vi "Initialize.vi"(0 "VISA resource name":refnum<visa-resource-name>, 1 "Error Queue Option":enum16{"Clear Error Queue", "Error Query"}(ring), 5 "RS-232 Settings":T1={"Read Term Char"=enum."CR", "Baud Rate"=enum."19200", "Flow Control\n(XON / XOFF)"=enum."Off"}, 7 "Instrument Type":T2=enum."KE6221", 11 "error in (no error)":errorcluster, 12 "ID Query? (T)":bool=TRUE, 13 "Reset? (T)":bool=TRUE) -> (4 "VISA resource name out":refnum<visa-resource-name>, 15 "error out":errorcluster)   [LabVIEW 2016, in "Keithley 622x.lvlib"]
doc: "Establishes communication with the instrument and optionally performs an instrument identification query and/or an instrument reset. Therefore, call this VI before calling other instrument driver VIs for this instrument. Generally, you need to call the Initialize VI only once at the beginning of an application."
uses:
  Keithley 622x.lvlib
  Utility/Typedefs/KE622x -- Instrument Type.ctl
  Utility/Typedefs/KE622x -- Serial Port Settings.ctl
panel:
  # "(c) 2010 Keithley Instruments.  ALL RIGHTS RESERVED."
  # "Serial settings must match those on the physical instrument.  Hardware flow control is not supported, but software flow control is (XON/XOFF)."
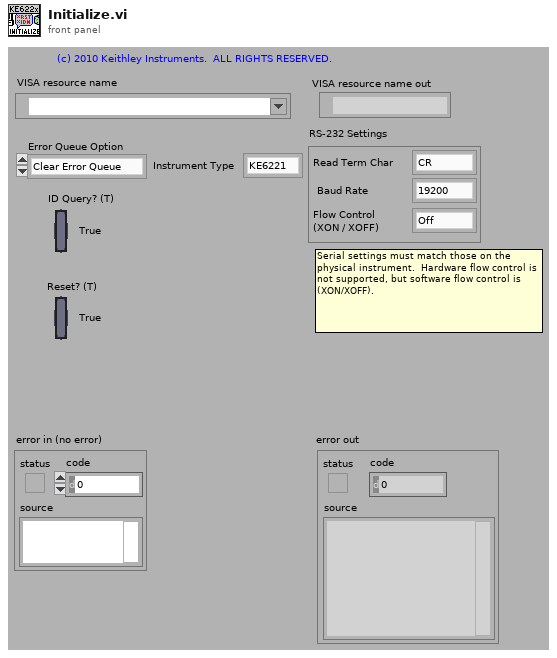
[diagram p1: front panel]
types:
  T1 = typedef "Keithley 622x.lvlib/KE622x -- Serial Port Settings.ctl" = cluster{"Read Term Char":enum16{"CR", "LF", "CR + LF", "LF + CR"}, "Baud Rate":enum16{"300", "600", "1200", "2400", "4800", "9600", "19200", "38400", "57600", "115200"}, "Flow Control\n(XON / XOFF)":enum16{"Off", "On"}}
  T2 = typedef "Keithley 622x.lvlib/KE622x -- Instrument Type.ctl" = enum16{"KE6220", "KE6221"}
  T3 = enum16{"300", "600", "1200", "2400", "4800", "9600", "19200", "38400", "57600", "115200"}
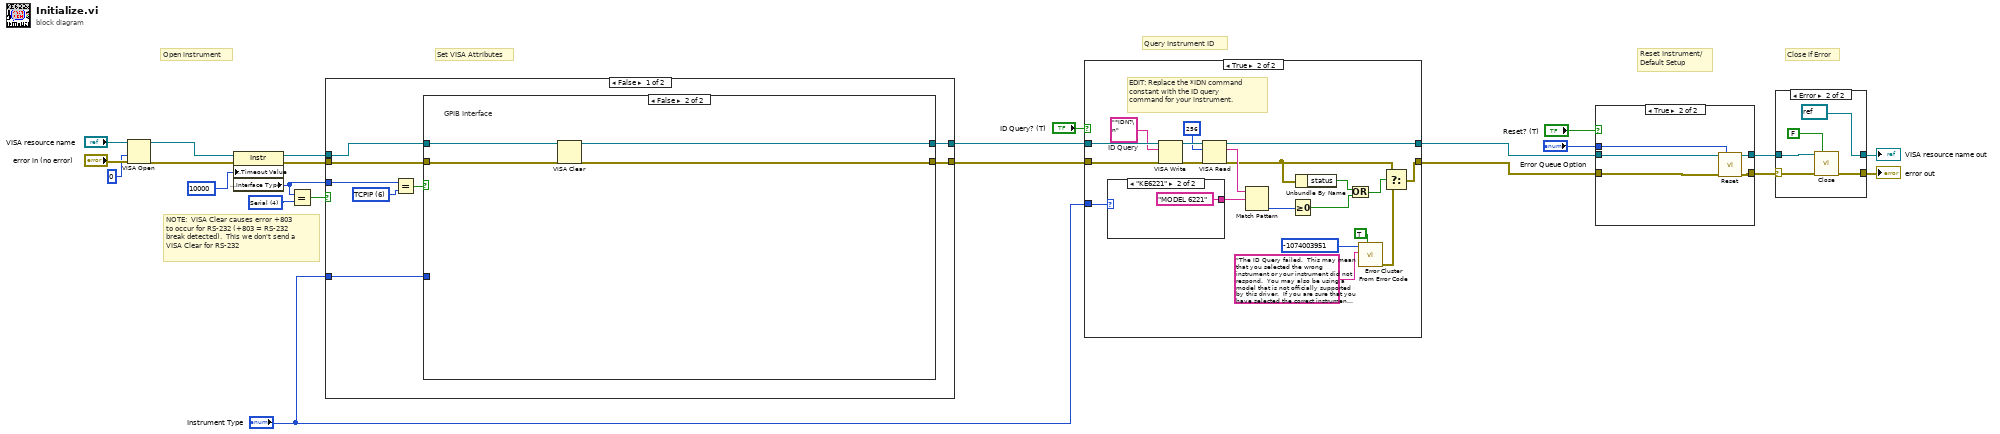
[diagram p0: block diagram]
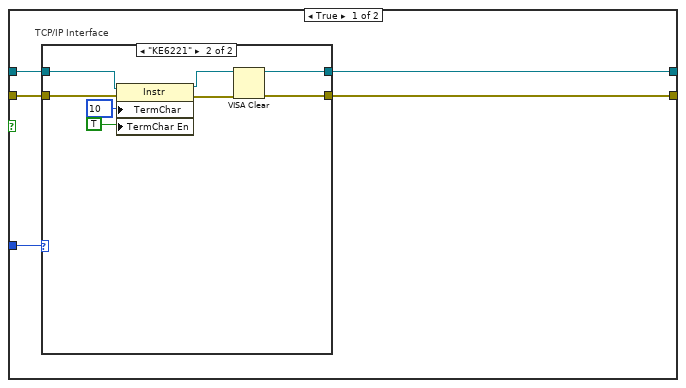
[diagram p2: hidden frame]
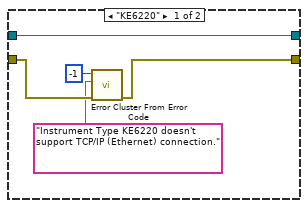
[diagram p3: hidden frame]
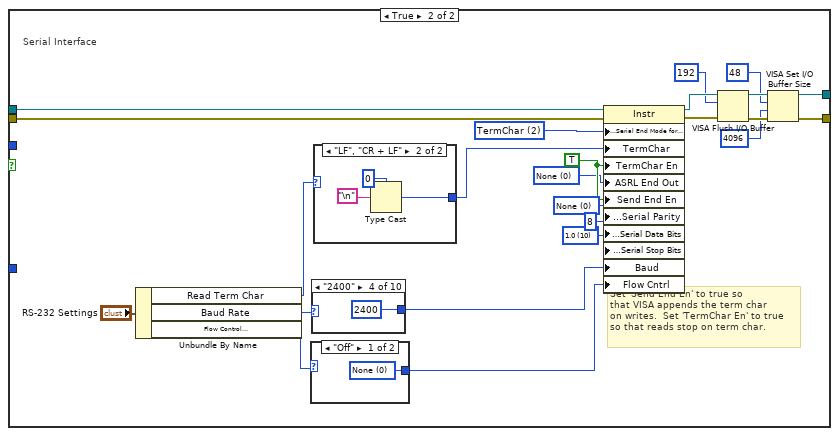
[diagram p4: hidden frame]
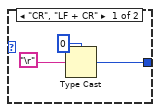
[diagram p5: hidden frame]
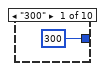
[diagram p6: hidden frame]
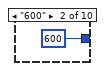
[diagram p7: hidden frame]
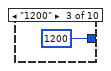
[diagram p8: hidden frame]
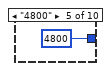
[diagram p9: hidden frame]
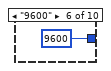
[diagram p10: hidden frame]
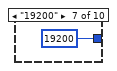
[diagram p11: hidden frame]
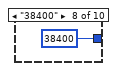
[diagram p12: hidden frame]
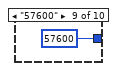
[diagram p13: hidden frame]
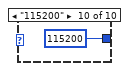
[diagram p14: hidden frame]
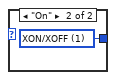
[diagram p15: hidden frame]
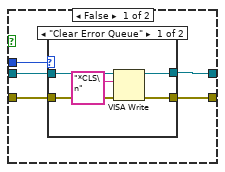
[diagram p17: hidden frame]
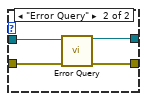
[diagram p18: hidden frame]
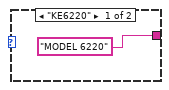
[diagram p20: hidden frame]
diagram:
  w11 = u16 4 items=["GPIB"=1, "VXI"=2, "GPIB-VXI"=3, "Serial"=4, "PXI"=5, "TCPIP"=6, "USB"=7] ("Interface Information:Interface Type")
  # "NOTE:  VISA Clear causes error +803\nto occur for RS-232 (+803 = RS-232\nbreak detected).  This we don't send a\nVISA Clear for RS-232"
  # "Set VISA Attributes"
  # "Close if Error"
  # "Query Instrument ID"
  # "Reset Instrument/\nDefault Setup"
  # "Open instrument"
  n1 = VISA Open(access mode=u32 0, error in (no error)="error in (no error)", VISA resource name="VISA resource name") -> (VISA resource name=w5:refnum<visa-resource-name>, error out=w4:errorcluster)  [unwired: 2 in]
  n2 = property class="Instr"(reference=w5, error in=w4, "General Settings:Timeout Value"=u32 10000) -> (reference out=w14:refnum<visa-resource-name>, error out=w13:errorcluster, "Interface Information:Interface Type"=w2:u16)
  n3 = Equal?(x=w2, y=w11) -> (x = y?=w12:bool)
  n4 = case shown="False" w12 {
    tunnel: [w28 w74] -> w16
    tunnel: [w29 w71] -> w15
    tunnel: w14 -> [w30 w76]
    tunnel: w13 -> [w31 w77]
    tunnel: w2 -> [w27 _]
    tunnel: "Instrument Type" -> [w24 _]
    frame False {
      w26 = u16 6 items=["GPIB"=1, "VXI"=2, "GPIB-VXI"=3, "Serial"=4, "PXI"=5, "TCPIP"=6, "USB"=7] ("Interface Information:Interface Type")
      n5 = Equal?(x=w27, y=w26) -> (x = y?=w25:bool)
      n6 = case shown="False" w25 {
        tunnel: w31 -> [w33 w50]
        tunnel: w30 -> [w34 w51]
        tunnel: [w36 w53] -> w29
        tunnel: [w35 w52] -> w28
        tunnel: w24 -> [w32 _]
        frame True {
          # "TCP/IP Interface"
          n7 = case shown="\"KE6221\"" w32 {
            tunnel: [w37 w49] -> w36
            tunnel: [w41 w48] -> w35
            tunnel: w34 -> [w41 w47]
            tunnel: w33 -> [w40 w44]
            frame "KE6220" {
              n8 = call <vilib>:"Error Cluster From Error Code.vi"("error in (no error)"=w40, "error message (\"\")"="Instrument Type KE6220 doesn't support TCP/IP (Ethernet) connection." ("error message (\"\")"), "error code (0)"=-1) -> ("error out"=w37:errorcluster)  [unwired: 6 in]
            }
            frame "KE6221" {
              n9 = property class="Instr"(reference=w47, error in=w44, "TermChar"=u8 10 ("Message Based Settings:Termination Character"), "TermChar En"=TRUE ("Message Based Settings:Termination Character Enable")) -> (reference out=w42:refnum<visa-resource-name>, error out=w43:errorcluster)
              n10 = VISA Clear(VISA resource name=w42, error in (no error)=w43) -> (VISA resource name out=w48:refnum<visa-resource-name>, error out=w49:errorcluster)
            }
          }
        }
        frame False {
          # "GPIB Interface"
          n11 = VISA Clear(VISA resource name=w51, error in (no error)=w50) -> (VISA resource name out=w52:refnum<visa-resource-name>, error out=w53:errorcluster)
        }
      }
    }
    frame True {
      w55 = u16 0 items=["None", "Last Bit", "TermChar", "Break"] ("Serial Settings:End Mode for Writes")
      w59 = u16 2 items=["None", "Last Bit", "TermChar"] ("Serial Settings:End Mode for Reads")
      w64 = u16 10 items=["1.0"=10, "1.5"=15, "2.0"=20] ("Serial Settings:Stop Bits")
      w66 = u16 0 items=["None", "Odd", "Even", "Mark", "Space"] ("Serial Settings:Parity")
      w58 = TRUE ("Message Based Settings:Termination Character Enable")
      # "Set 'Send End En' to true so\nthat VISA appends the term char\non writes.  Set 'TermChar En' to true\nso that reads stop on term char."
      # "Serial Interface"
      n12 = Unbundle By Name("RS-232 Settings") -> ("Read Term Char"=w61:enum16{"CR", "LF", "CR + LF", "LF + CR"}, "Baud Rate"=w62:T3, "Flow Control\n(XON / XOFF)"=w63:enum16{"Off", "On"})
      n13 = case shown="\"Off\"" w63 {
        tunnel: [w94 w95] -> w56
        frame "Off" {
          w94 = u16 0 items=["None", "XON/XOFF", "RTS/CTS", "XON/XOFF & RTS/CTS", "DTR/DSR", "XON/XOFF & DTR/DSR"] ("Serial Settings:Flow Control")
        }
        frame "On" {
          w95 = u16 1 items=["None", "XON/XOFF", "RTS/CTS", "XON/XOFF & RTS/CTS", "DTR/DSR", "XON/XOFF & DTR/DSR"] ("Serial Settings:Flow Control")
        }
      }
      n14 = case shown="\"2400\"" w62 {
        tunnel: [u32 300 ("Serial Settings:Baud Rate") u32 600 ("Serial Settings:Baud Rate") u32 1200 ("Serial Settings:Baud Rate") u32 2400 ("Serial Settings:Baud Rate") u32 4800 ("Serial Settings:Baud Rate") u32 9600 ("Serial Settings:Baud Rate") u32 19200 ("Serial Settings:Baud Rate") u32 38400 ("Serial Settings:Baud Rate") u32 57600 ("Serial Settings:Baud Rate") u32 115200 ("Serial Settings:Baud Rate")] -> w57
        frame "300" {
        }
        frame "600" {
        }
        frame "1200" {
        }
        frame "2400" {
        }
        frame "4800" {
        }
        frame "9600" {
        }
        frame "19200" {
        }
        frame "38400" {
        }
        frame "57600" {
        }
        frame "115200" {
        }
      }
      n15 = case shown="\"LF\", \"CR + LF\"" w61 {
        tunnel: [w78 w82] -> w60
        frame "CR", "LF + CR" {
          n16 = Type Cast(type=u8 0, x="\r") -> (*(type *) &x=w78:u8)
        }
        frame "LF", "CR + LF" {
          n17 = Type Cast(type=u8 0, x="\n") -> (*(type *) &x=w82:u8)
        }
      }
      n18 = property class="Instr"(reference=w76, error in=w77, "Serial Settings:Serial End Mode for Reads"=w59, "TermChar"=w60, "TermChar En"=w58, "ASRL End Out"=w55, "Send End En"=w58, "Serial Settings:Serial Parity"=w66, "Serial Settings:Serial Data Bits"=u16 8 ("Serial Settings:Data Bits"), "Serial Settings:Serial Stop Bits"=w64, "Baud"=w57, "Flow Cntrl"=w56) -> (reference out=w70:refnum<visa-resource-name>, error out=w73:errorcluster)
      n19 = VISA Flush I/O Buffer(VISA resource name=w70, mask (16)=u16 192, error in (no error)=w73) -> (VISA resource name out=w75:refnum<visa-resource-name>, error out=w72:errorcluster)
      n20 = VISA Set I/O Buffer Size(VISA resource name=w75, mask (16)=u16 48, size (4096)=u32 4096 ("size (0)"), error in (no error)=w72) -> (VISA resource name out=w74:refnum<visa-resource-name>, error out=w71:errorcluster)
    }
  }
  n21 = case shown="True" "ID Query? (T)" {
    tunnel: [w96 w117] -> w22
    tunnel: [w97 w114] -> w23
    tunnel: w16 -> [w97 w115]
    tunnel: w15 -> [w96 w116]
    tunnel: "Instrument Type" -> [_ w99]
    frame False {
    }
    frame True {
      w109 = "*IDN?\n"  # ID Query
      # "EDIT: Replace the *IDN command\nconstant with the ID query\ncommand for your instrument."
      n22 = case shown="\"KE6221\"" w99 {
        tunnel: ["MODEL 6220" "MODEL 6221"] -> w98
        frame "KE6220" {
        }
        frame "KE6221" {
        }
      }
      n23 = VISA Write(VISA resource name=w115, write buffer=w109, error in (no error)=w116) -> (VISA resource name out=w112:refnum<visa-resource-name>, error out=w111:errorcluster)  [unwired: 1 out]
      n24 = VISA Read(VISA resource name=w112, byte count=u32 256, error in (no error)=w111) -> (VISA resource name out=w114:refnum<visa-resource-name>, read buffer=w113:string, error out=w103:errorcluster)  [unwired: 1 out]
      n25 = Match Pattern(string=w113, regular expression=w98) -> (offset past match=w104:i32)  [unwired: 1 in, 3 out]
      n26 = Greater Or Equal To 0?(x=w104) -> (x >= 0?=w101:bool)
      n27 = Unbundle By Name(w103) -> ("status"=w102:bool)
      n28 = Or(x=w102, y=w101) -> (x .or. y?=w100:bool)
      n29 = call <vilib>:"Error Cluster From Error Code.vi"("show call chain? (False)"=TRUE, "error message (\"\")"="The ID Query failed.  This may mean that you selected the wrong instrument or your instrument did not respond.  You may also be using a model that is not officially supported by this driver.  If you are sure that you have selected the correct instrument and it is responding, try disabling the ID Query." ("Source (VI Name)"), "error code (0)"=-1074003951 ("Code")) -> ("error out"=w108:errorcluster)  [unwired: 6 in]
      n30 = Select(t=w103, s=w100, f=w108) -> (s? t:f=w117:errorcluster)
    }
  }
  n31 = case shown="True" "Reset? (T)" {
    tunnel: w22 -> [w121 w137]
    tunnel: [w123 w136] -> w6
    tunnel: w23 -> [w122 w138]
    tunnel: [w124 w135] -> w7
    tunnel: "Error Queue Option" -> [w120 w134]
    frame False {
      n32 = case shown="\"Clear Error Queue\"" w120 {
        tunnel: [w126 w133] -> w124
        tunnel: [w127 w132] -> w123
        tunnel: w122 -> [w129 w131]
        tunnel: w121 -> [w128 w130]
        frame "Clear Error Queue" {
          n33 = VISA Write(VISA resource name=w129, write buffer="*CLS\n", error in (no error)=w128) -> (VISA resource name out=w126:refnum<visa-resource-name>, error out=w127:errorcluster)  [unwired: 1 out]
        }
        frame "Error Query" {
          n34 = call "Error Query.vi"("VISA Resource In"=w131, "error in (no error)"=w130) -> ("VISA Resource Out (dupl)"=w133:refnum<visa-resource-name>, "error out"=w132:errorcluster)  [unwired: 10 in, 2 out]
        }
      }
    }
    frame True {
      n35 = call "Reset.vi"("VISA resource name"=w138, "Error Queue Option"=w134, "error in (no error)"=w137) -> ("VISA resource name out"=w135:refnum<visa-resource-name>, "error out"=w136:errorcluster)  [unwired: 11 in]
    }
  }
  n36 = case shown="Error" w6 {
    selector: w6 -> [w139 w143]
    tunnel: w7 -> [w140 w144]
    tunnel: [w140 refnum<visa-resource-name> refnum ("VISA resource name out")] -> w9
    tunnel: [w139 w145] -> w8
    frame No Error {
    }
    frame Error {
      n37 = call "Close.vi"("VISA resource name"=w144, "Query For SCPI Errors? (T)"=FALSE, "error in (no error)"=w143) -> ("error out"=w145:errorcluster)  [unwired: 12 in]
    }
  }
  "VISA resource name out" <- w9
  "error out" <- w8
